vi "sub_UnionOfValidIndexes.vi"(8 "error in (no error)":errorcluster, 10 "set 2":string[](array[string]), 11 "set 1":string[](array[string])) -> (0 "error out":errorcluster, 3 "set 1  & set 2":string[](array[string]))   [LabVIEW 2018]
panel:
  # "returns the union of set 1 and set 2"
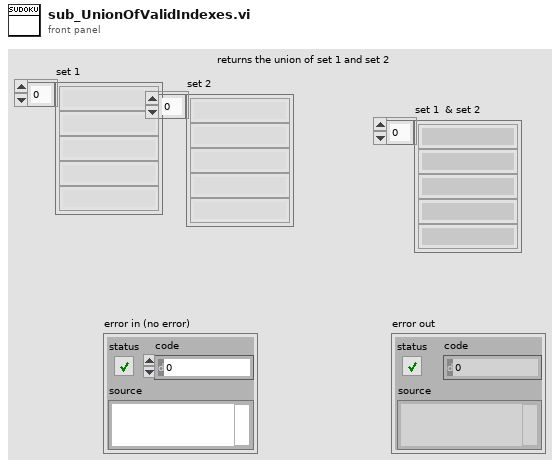
[diagram p1: front panel]
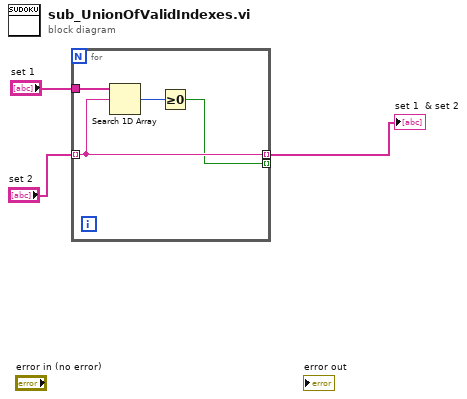
[diagram p0: block diagram]
diagram:
  n1 = for {
    tunnel: "set 1" -> [w7]
    tunnel: "set 2" -> [w5] mode=indexing
    tunnel: [w5] -> w1 mode=indexing if=w4
    tunnel: [w4] -> _ mode=indexing
    n2 = Search 1D Array(1D array=w7, element=w5) -> (index of element=w6:i32)  [unwired: 1 in]
    n3 = Greater Or Equal To 0?(x=w6) -> (x >= 0?=w4:bool)
  }
  "set 1  & set 2" <- w1
